vi "SLL DE DI Driver.vi"(7 "DI Driver Option":T2, 8 "error in (no error)":errorcluster, 10 "AI Channel Name Array":T1[](array[typedef]), 11 "AI Channel Name":T1) -> (0 "error out":errorcluster, 2 "DI Channel Value Array":bool[](array[boolean]), 3 "DI Channel Value":bool)   [LabVIEW 2013]
doc: "Copyright © 2005, Soliton Technologies.\nAll rights reserved."
uses:
  Controls/SLL DE DI Global Options.ctl
  Controls/SLL DE List of Digital Inputs.ctl
  Controls/SLL DE DAQ Global Options.ctl
  Controls/SLL DE DAQ Global Elements.ctl
  <vilib>/DAQmx/read.llb/DAQmx Read (Digital Bool 1Line 1Point).vi
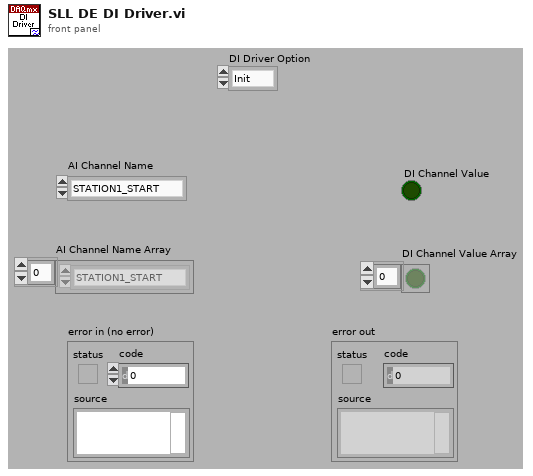
[diagram p1: front panel]
types:
  T1 = typedef "SLL DE List of Digital Inputs.ctl" = enum16{"STATION1_START", "STATION1_STOP", "STATION1_CLAMPED", "STATION1_TC_PASS", "STATION1_TC_FAIL", "STATION1_TTA", "STATION1_TTB", "STATION2_START", "STATION2_STOP", "STATION2_CLAMPED", "STATION2_TC_PASS", "STATION2_TC_FAIL", "STATION2_TTA", "STATION2_TTB", "STATION3_START", "STATION3_STOP", "STATION3_CLAMPED", "STATION3_TC_PASS", "STATION3_TC_FAIL", "STATION3_TTA", "STATION3_TTB", "STATION4_START", "STATION4_STOP", "STATION4_CLAMPED", "STATION4_TC_PASS", "STATION4_TC_FAIL", "STATION4_TTA", "STATION4_TTB"}
  T2 = typedef "SLL DE DI Global Options.ctl" = enum16{"Init", "Write Line", "Write Array", "Read Line", "Read Array", "Read Full Status", "Write Full Status"}
  T3 = typedef "SLL DE DAQ Global Elements.ctl" = enum16{"AI Error", "AO Error", "DI Error", "DO Error", "AI Restart", "DI Restart", "AI Running", "AO Running", "DI Running", "DO Running", "DAQ Exit?"}
  T4 = typedef "SLL DE DAQ Global Options.ctl" = enum16{"Init", "Write 1", "Read 1", "Write Array", "Read Array", "Clear"}
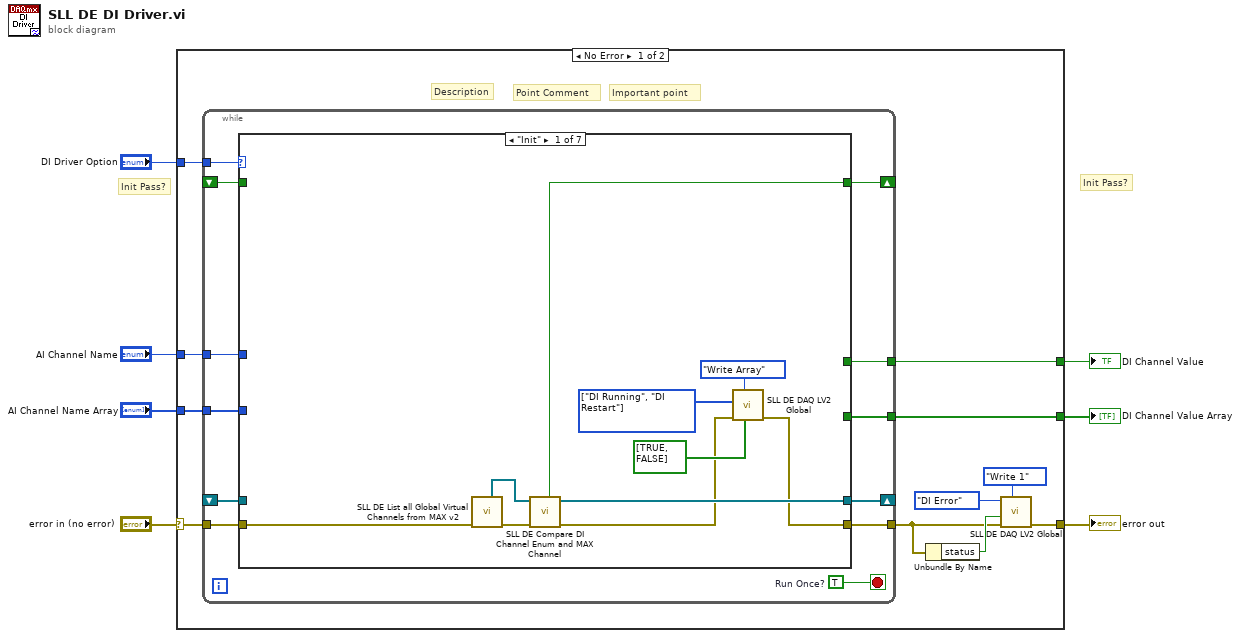
[diagram p0: block diagram]
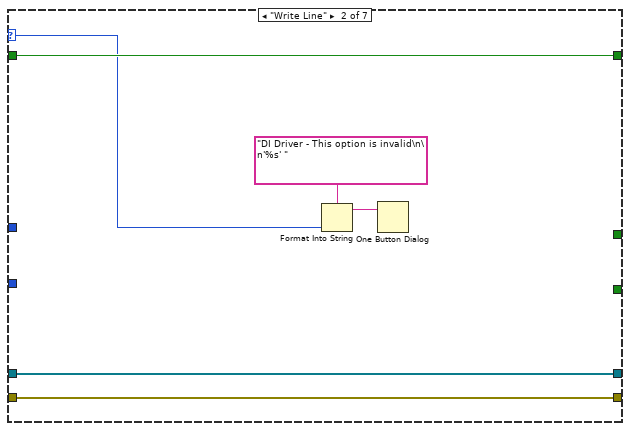
[diagram p2: hidden frame]
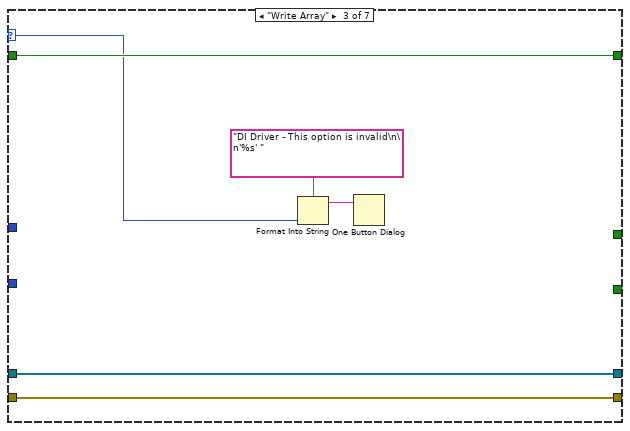
[diagram p3: hidden frame]
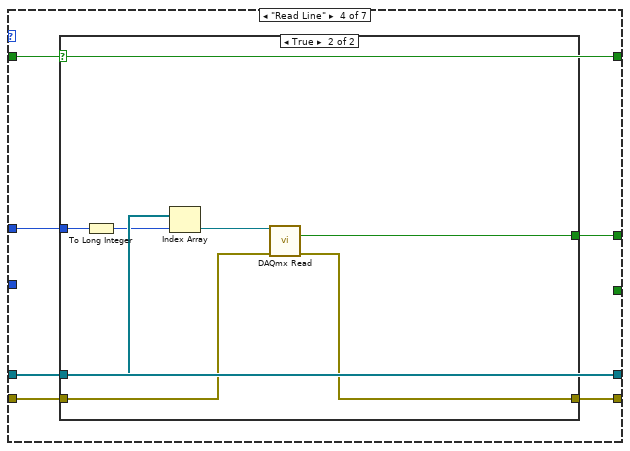
[diagram p4: hidden frame]
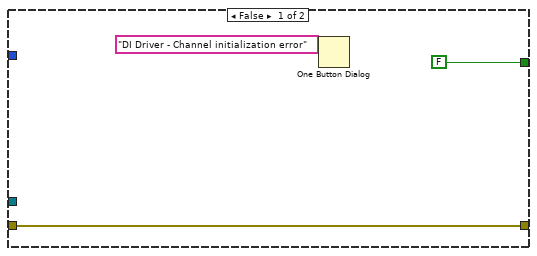
[diagram p5: hidden frame]
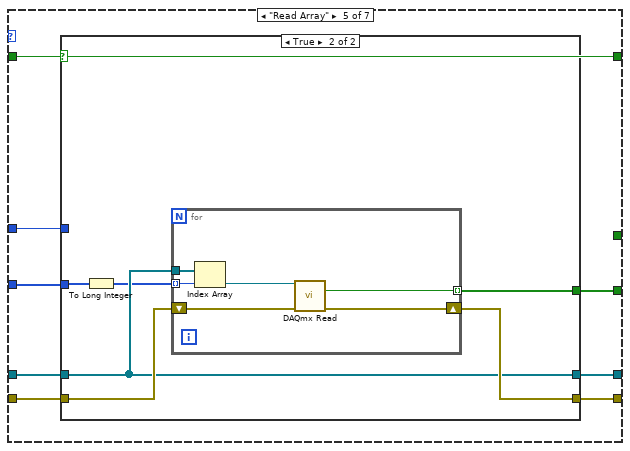
[diagram p6: hidden frame]
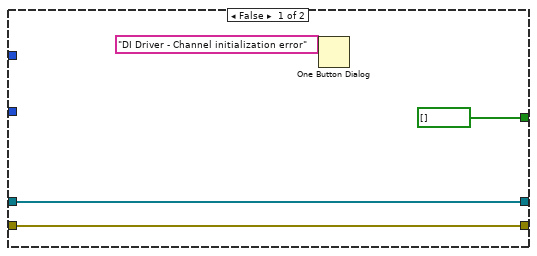
[diagram p7: hidden frame]
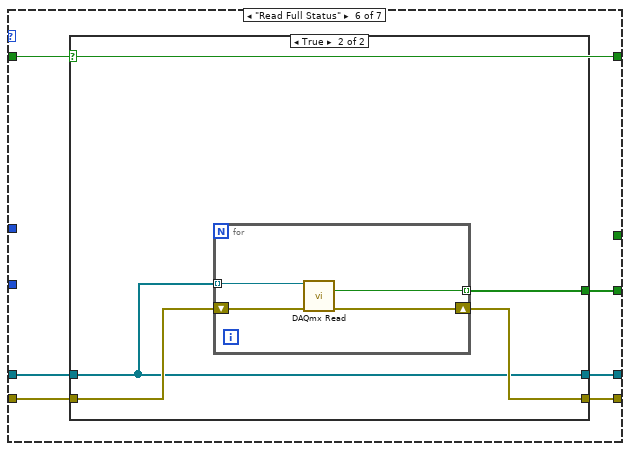
[diagram p8: hidden frame]
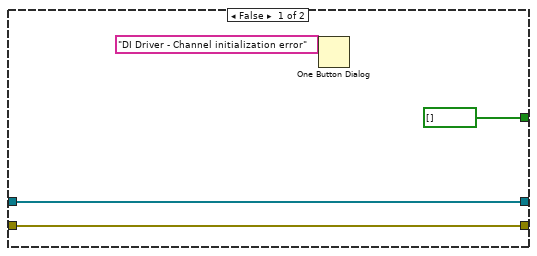
[diagram p9: hidden frame]
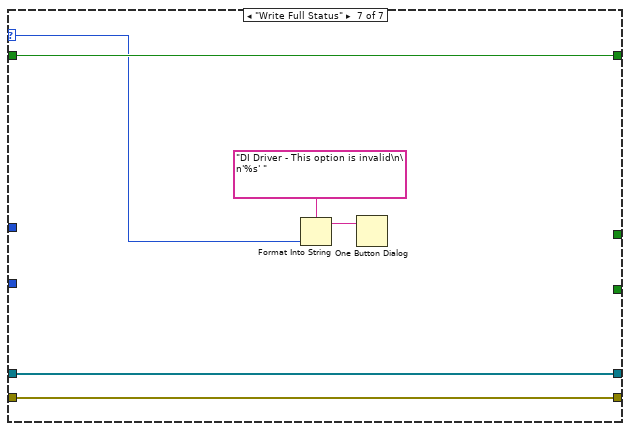
[diagram p10: hidden frame]
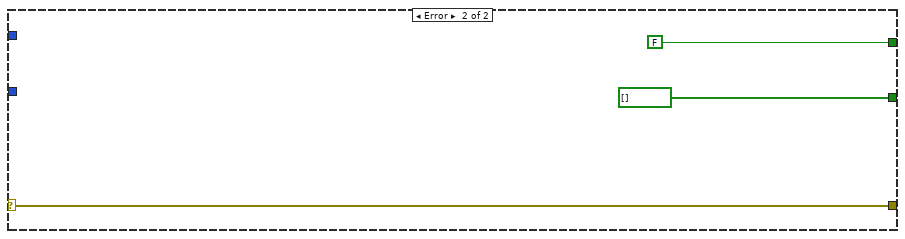
[diagram p11: hidden frame]
diagram:
  # "Init Pass?"
  # "Init Pass?"
  n1 = case shown="No Error" "error in (no error)" {
    selector: "error in (no error)" -> [w18 w119]
    tunnel: [w8 w119] -> w6
    tunnel: "DI Driver Option" -> [w17 _]
    tunnel: "AI Channel Name" -> [w16 _]
    tunnel: [w15 FALSE] -> w3
    tunnel: "AI Channel Name Array" -> [w14 _]
    tunnel: [w13 bool[] []] -> w1
    frame No Error {
      # "Point Comment"
      # "Important point"
      # "Description"
      n2 = while {
        tunnel: w18 -> [w29]
        tunnel: [w28] -> w9
        shift-right: [w27] -> _
        shift-left: _ -> [w24]
        shift-right: [w26] -> _
        shift-left: _ -> [w23]
        tunnel: w17 -> [w25]
        tunnel: w16 -> [w22]
        tunnel: [w21] -> w15
        tunnel: w14 -> [w20]
        tunnel: [w19] -> w13
        stop <- w30 stop-if-true
        w30 = TRUE  # Run Once?
        n3 = case shown="\"Init\"" w25 {
          selector: w25 -> [_ w41 w47 _ _ _ w111]
          tunnel: w29 -> [w39 w44 w50 w56 w76 w98 w115]
          tunnel: [w31 w44 w50 w55 w73 w94 w115] -> w28
          tunnel: [w37 w46 w52 w53 w69 w93 w116] -> w27
          tunnel: [w38 w45 w51 w58 w72 w95 w114] -> w26
          tunnel: w24 -> [_ w46 w52 w53 w69 w93 w116]
          tunnel: w23 -> [_ w45 w51 w58 w75 w97 w114]
          tunnel: w22 -> [_ _ _ w57 w74 _ _]
          tunnel: [_ _ _ w54 _ _ _] -> w21
          tunnel: w20 -> [_ _ _ _ w71 _ _]
          tunnel: [_ _ _ _ w70 w96 _] -> w19
          frame "Init" {
            w34 = T3[] [enum."DI Running", enum."DI Restart"] items=["AI Error", "AO Error", "DI Error", "DO Error", "AI Restart", "DI Restart", "AI Running", "AO Running", "DI Running", "DO Running", "DAQ Exit?"] ("Elements Array")
            n4 = call "SLL DE List all Global Virtual Channels from MAX v2.vi"("error in (no error)"=w39) -> ("error out"=w40:errorcluster, "Digital Input"=w36:refnum<k21>[])  [unwired: 4 in, 5 out]
            n5 = call "SLL DE Compare DI Channel Enum and MAX Channel.vi"("error in (no error)"=w40, "Digital Input Channels"=w36) -> ("error out"=w32:errorcluster, "Channels Out"=w38:refnum<k21>[], "Pass?"=w37:bool)  [unwired: 7 in]
            n6 = call "SLL DE DAQ LV2 Global.vi"("Status Array In"=bool[] [TRUE, FALSE], "Option"=SLL_DE_DAQ_Global_Options."Write Array", "error in (no error)"=w32, "Elements Array"=w34) -> ("error out"=w31:errorcluster)  [unwired: 5 in, 2 out]
          }
          frame "Write Line" {
            n7 = Format Into String(format string="DI Driver - This option is invalid\n\n'%s' " ("message"), w41) -> (resulting string=w42:string)  [unwired: 2 in, 1 out]
            n8 = One Button Dialog(message=w42) -> ()  [unwired: 1 in, 1 out]
          }
          frame "Write Array" {
            n9 = Format Into String(format string="DI Driver - This option is invalid\n\n'%s' " ("message"), w47) -> (resulting string=w48:string)  [unwired: 2 in, 1 out]
            n10 = One Button Dialog(message=w48) -> ()  [unwired: 1 in, 1 out]
          }
          frame "Read Line" {
            n11 = case shown="True" w53 {
              tunnel: w58 -> [_ w68]
              tunnel: w57 -> [_ w67]
              tunnel: w56 -> [w60 w64]
              tunnel: [w60 w63] -> w55
              tunnel: [FALSE w62] -> w54
              frame False {
                n12 = One Button Dialog(message="DI Driver - Channel initialization error") -> ()  [unwired: 1 in, 1 out]
              }
              frame True {
                n13 = To Long Integer(number=w67) -> (32bit integer=w66:i32)
                n14 = Index Array(array=w68, index=w66) -> (element=w65:refnum<k21>)
                n15 = call-poly <vilib>:"DAQmx Read.vi"("task/channels in"=w65, "error in"=w64) -> ("data"=w62:bool, "error out"=w63:errorcluster)  [unwired: 11 in, 1 out]
              }
            }
          }
          frame "Read Array" {
            n16 = case shown="True" w69 {
              tunnel: w75 -> [w78 w83]
              tunnel: w74 -> [_ _]
              tunnel: w76 -> [w80 w86]
              tunnel: [w80 w85] -> w73
              tunnel: [bool[] [] w84] -> w70
              tunnel: [w78 w83] -> w72
              tunnel: w71 -> [_ w82]
              frame False {
                n17 = One Button Dialog(message="DI Driver - Channel initialization error") -> ()  [unwired: 1 in, 1 out]
              }
              frame True {
                n18 = To Long Integer(number=w82) -> (32bit integer=w81:i32[])
                n19 = for {
                  tunnel: w81 -> [w92] mode=indexing
                  tunnel: [w87] -> w84 mode=indexing
                  tunnel: w83 -> [w88]
                  shift-right: [w89] -> w85
                  shift-left: w86 -> [w90]
                  n20 = Index Array(array=w88, index=w92) -> (element=w91:refnum<k21>)
                  n21 = call-poly <vilib>:"DAQmx Read.vi"("task/channels in"=w91, "error in"=w90) -> ("data"=w87:bool, "error out"=w89:errorcluster)  [unwired: 11 in, 1 out]
                }
              }
            }
          }
          frame "Read Full Status" {
            n22 = case shown="True" w93 {
              tunnel: w97 -> [w100 w103]
              tunnel: w98 -> [w102 w106]
              tunnel: [w102 w105] -> w94
              tunnel: [bool[] [] w104] -> w96
              tunnel: [w100 w103] -> w95
              frame False {
                n23 = One Button Dialog(message="DI Driver - Channel initialization error") -> ()  [unwired: 1 in, 1 out]
              }
              frame True {
                n24 = for {
                  tunnel: [w107] -> w104 mode=indexing
                  tunnel: w103 -> [w108] mode=indexing
                  shift-right: [w109] -> w105
                  shift-left: w106 -> [w110]
                  n25 = call-poly <vilib>:"DAQmx Read.vi"("task/channels in"=w108, "error in"=w110) -> ("data"=w107:bool, "error out"=w109:errorcluster)  [unwired: 11 in, 1 out]
                }
              }
            }
          }
          frame "Write Full Status" {
            n26 = Format Into String(format string="DI Driver - This option is invalid\n\n'%s' " ("message"), w111) -> (resulting string=w112:string)  [unwired: 2 in, 1 out]
            n27 = One Button Dialog(message=w112) -> ()  [unwired: 1 in, 1 out]
          }
        }
      }
      n28 = Unbundle By Name(w9) -> ("status"=w10:bool)
      n29 = call "SLL DE DAQ LV2 Global.vi"("Option"=SLL_DE_DAQ_Global_Options."Write 1", "error in (no error)"=w9, "Status In"=w10, "Element"=SLL_DE_DAQ_Global_Elements."DI Error") -> ("error out"=w8:errorcluster)  [unwired: 5 in, 2 out]
    }
    frame Error {
    }
  }
  "error out" <- w6
  "DI Channel Value" <- w3
  "DI Channel Value Array" <- w1
